vi "Teleop.vi"(10 "Match Info":T1={"Autonomous Elapsed Seconds"=0.0, "TeleOp Elapsed Seconds"=0.0, "Disabled Elapsed Seconds"=0.0, "Visited Autonomous"=FALSE, "Visited TeleOp"=FALSE, "Visited Disabled"=FALSE, "Autonomous Settings"={"Autonomous Style"=enum."Independent", "VI Refnum"=refnum}}, 11 "Call Context":T2) -> ()   [LabVIEW 2013]
doc: "This VI is called for each TeleOp packet received from the DS where the robot is not disabled. It is often used to read from the joysticks and update I/O or to update setpoints for timed control loops. It should complete and return within 20 milliseconds or it may miss DS packets."
uses:
  <vilib>/Rock Robotics/WPI/DriverStation/WPI_DriverStationDerivedRobotMode.ctl
  <vilib>/Rock Robotics/WPI/DriverStation/WPI_DriverStationMatch Info.ctl
  Robot Global Data.vi
  <vilib>/Rock Robotics/WPI/Joystick/WPI_JoystickGetSetRefNum.vi
  <vilib>/Rock Robotics/WPI/RobotDrive/WPI_RobotDriveGetSetRefNum.vi
panel:
  out "Numeric 1":dbl(slide) scale=0.0..100.0
  out "Boolean 2":bool
  out "Boolean 1":bool
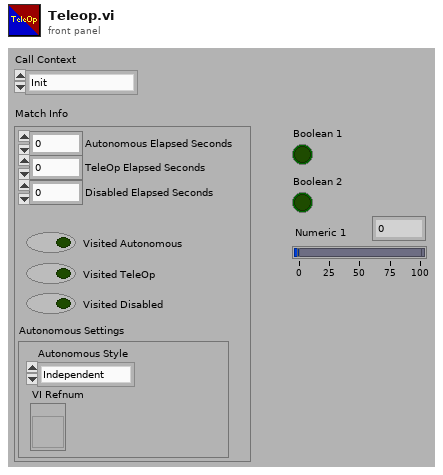
[diagram p1: front panel]
types:
  T1 = typedef "WPI_DriverStationMatch Info.ctl" = cluster{"Autonomous Elapsed Seconds":dbl, "TeleOp Elapsed Seconds":dbl, "Disabled Elapsed Seconds":dbl, "Visited Autonomous":bool, "Visited TeleOp":bool, "Visited Disabled":bool, "Autonomous Settings":cluster{"Autonomous Style":enum16{"Iterative", "Independent"}, "VI Refnum":refnum<vi>}}
  T2 = typedef "WPI_DriverStationDerivedRobotMode.ctl" = enum16{"Init", "Execute", "Stop"}
  T3 = typedef "WPI_JoystickDevRef.ctl" = cluster{"Device":T4}
  T4 = typedef "WPI_JoystickDeviceEnum.ctl" = enum16{"USB 1", "USB 2", "USB 3", "USB 4", "Kinect 1", "Kinect 2"}
  T5 = typedef "WPI_JoystickButtonState.ctl" = cluster{"Button 1":bool, "Button 2":bool, "Button 3":bool, "Button 4":bool, "Button 5":bool, "Button 6":bool, "Button 7":bool, "Button 8":bool, "Button 9":bool, "Button 10":bool, "Button 11":bool, "Button 12":bool}
  T6 = cluster{"axis 1 (x)":dbl, "axis 2 (y)":dbl, "axis 3 (throttle)":dbl, "axis 4":dbl, "axis 5":dbl, "axis 6":dbl}
  T7 = typedef "WPI_RobotDriveDevRef.ctl" = cluster{"DevStatus":errorcluster, "Motors[]":T8[], "Square Inputs":bool, "Max Output":dbl, "Isochronous":bool}
  T8 = typedef "WPI_MotorControlDeviceRef.ctl" = cluster{"DeviceStatus":errorcluster, "Type":enum16{"PWM", "CAN"}, "PWM":cluster{"Digital Module":T9, "PWM Channel":T10, "DeadBand":T11}, "CAN":cluster{"Device Number":u8, "Control Mode":T12, "Semaphore":T13, "Max Vout":dbl}, "Invert":bool, "TransformRef":T14, "InvTransformRef":T14}
  T9 = typedef "FPGA_TypedefDigitalModule.ctl" = enum16{"Digital Module 1", "Digital Module 2"}
  T10 = typedef "FPGA_DIOPWMChannel.ctl" = enum8{"PWM 1", "PWM 2", "PWM 3", "PWM 4", "PWM 5", "PWM 6", "PWM 7", "PWM 8", "PWM 9", "PWM 10", "Invalid"}
  T11 = typedef "WPI_PWMDeadband.ctl" = cluster{"Name":string, "maxPositivePwm":i32, "minPositivePwm":i32, "centerPwm":i32, "maxNegativePwm":i32, "minNegativePwm":i32, "angularRange":u16}
  T12 = typedef "WPI_CANJaguar_ControlMode.ctl" = enum8{"Percent VBus", "Current", "Speed", "Position", "Voltage"}
  T13 = typedef "Semaphore RefNum" = refnum<k1>
  T14 = typedef "WPI_PWMTransform_ConPane.ctl" = refnum<vi>
  T15 = typedef "WPI_ServoDeviceRef.ctl" = cluster{"DeviceStatus":errorcluster, "Digital Module":T9, "PWM Channel":T10, "DeadBand":T11}
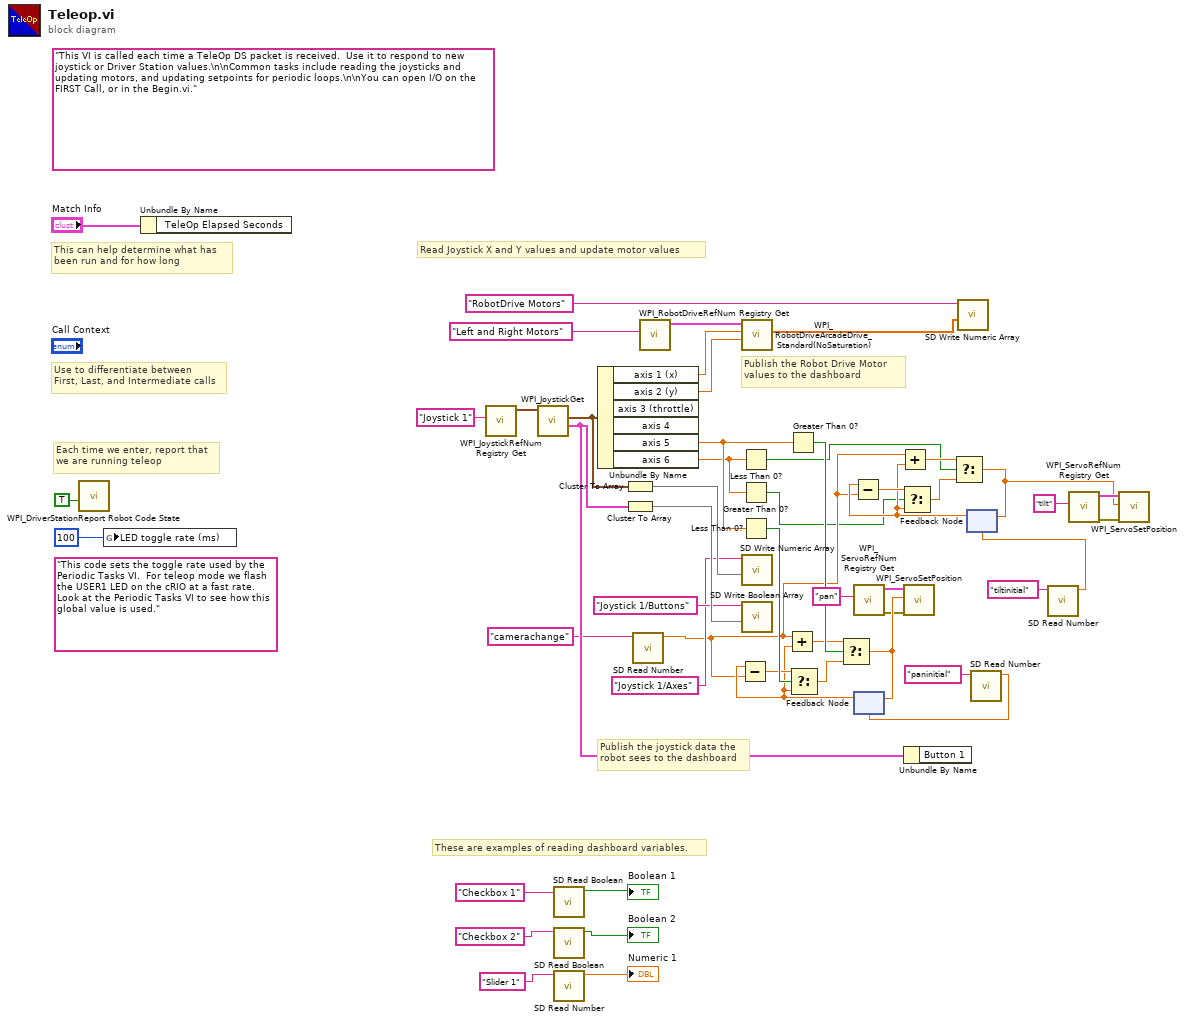
[diagram p0: block diagram]
diagram:
  (unwired) "This code sets the toggle rate used by the Periodic Tasks VI.  For teleop mode we flash the USER1 LED on the cRIO at a fast rate.  Look at the Periodic Tasks VI to see how this global value is used."
  (unwired) "This VI is called each time a TeleOp DS packet is received.  Use it to respond to new joystick or Driver Station values.\n\nCommon tasks include reading the joysticks and updating motors, and updating setpoints for periodic loops.\n\nYou can open I/O on the FIRST Call, or in the Begin.vi."
  # "These are examples of reading dashboard variables."
  # "Publish the Robot Drive Motor\nvalues to the dashboard"
  # "Publish the joystick data the\nrobot sees to the dashboard"
  # "Each time we enter, report that\nwe are running teleop"
  # "Use to differentiate between\nFirst, Last, and Intermediate calls"
  # "This can help determine what has\nbeen run and for how long"
  # "Read Joystick X and Y values and update motor values"
  n1 = call <vilib>:"WPI_DriverStationReport Robot Code State.vi"("TeleOp"=TRUE ("Autonomous")) -> ()  [unwired: 10 in, 1 out]
  n2 = global write "Robot Global Data.vi" "LED toggle rate (ms)"(u32 100 ("LED ms toggle rate")) -> ()
  n3 = Unbundle By Name("Match Info") -> ()  [unwired: 1 out]
  n4 = call <vilib>:"WPI_JoystickRefNum Registry Get.vi"("refnum name"="Joystick 1") -> ("JoystickDevRef"=w45:T3)  [unwired: 1 in, 9 out]
  n5 = call <vilib>:"WPI_JoystickGet.vi"("JoystickDevRef"=w45) -> ("Buttons"=w29:T5, "Axes"=w40:T6)  [unwired: 1 in, 4 out]
  n6 = call <vilib>:"SD Read Boolean.vi"("Name"="Checkbox 1" ("refnum name")) -> ("Boolean"=→"Boolean 1":bool)  [unwired: 8 in, 2 out]
  n7 = call <vilib>:"SD Read Boolean.vi"("Name"="Checkbox 2" ("refnum name")) -> ("Boolean"=→"Boolean 2":bool)  [unwired: 8 in, 2 out]
  n8 = call <vilib>:"SD Read Number.vi"("Name"="Slider 1" ("refnum name")) -> ("Numeric"=→"Numeric 1":dbl)  [unwired: 8 in, 2 out]
  n9 = Unbundle By Name(w40) -> ("axis 1 (x)"=w48:dbl, "axis 2 (y)"=w47:dbl, "axis 5"=w28:dbl, "axis 6"=w27:dbl)  [unwired: 2 out]
  n10 = Cluster To Array(cluster=w40) -> (array=w39:dbl[])
  n11 = Cluster To Array(cluster=w29) -> (array=w42:bool[])
  n12 = call <vilib>:"SD Read Number.vi"("Name"="camerachange") -> ("Numeric"=w8:dbl)  [unwired: 8 in, 2 out]
  n13 = call <vilib>:"WPI_RobotDriveRefNum Registry Get.vi"("refnum name"="Left and Right Motors") -> ("RobotDriveDevRef"=w49:T7)  [unwired: 1 in, 9 out]
  n14 = Less Than 0?(x=w27) -> (x < 0?=w7:bool)
  n15 = Greater Than 0?(x=w27) -> (x > 0?=w6:bool)
  n16 = Less Than 0?(x=w28) -> (x < 0?=w25:bool)
  n17 = call <vilib>:"WPI_RobotDriveArcadeDrive_Standard(NoSaturation).vi"("Y axis value"=w47, "X axis value"=w48, "RobotDriveDevRef"=w49) -> ("Motor Values"=w36:dbl[])  [unwired: 1 in, 7 out]
  n18 = call <vilib>:"SD Write Numeric Array.vi"("Numeric Array"=w39, "Name"="Joystick 1/Axes") -> ()  [unwired: 8 in, 2 out]
  n19 = call <vilib>:"SD Write Boolean Array.vi"("Boolean Array"=w42, "Name"="Joystick 1/Buttons") -> ()  [unwired: 8 in, 2 out]
  n20 = Greater Than 0?(x=w28) -> (x > 0?=w24:bool)
  n21 = call <vilib>:"WPI_ServoRefNum Registry Get.vi"("refnum name"="pan") -> ("error out"=w16:errorcluster, "ServoDeviceRef"=w17:T15)  [unwired: 9 in]
  n22 = Unbundle By Name(w29) -> ()  [unwired: 1 out]
  n23 = call <vilib>:"SD Write Numeric Array.vi"("Numeric Array"=w36, "Name"="RobotDrive Motors") -> ()  [unwired: 8 in, 2 out]
  n24 = call <vilib>:"SD Read Number.vi"("Name"="paninitial") -> ("Numeric"=w3:dbl)  [unwired: 8 in, 2 out]
  n25 = feedback #1(w3) -> (w19:dbl)
  n26 = Subtract(x=w19, y=w8) -> (x-y=w21:dbl)
  n27 = Add(x=w8, y=w19) -> (x+y=w20:dbl)
  n28 = Select(t=w21, s=w25, f=w19) -> (s? t:f=w22:dbl)
  n29 = Select(t=w20, s=w24, f=w22) -> (s? t:f=w23:dbl)
  n30 = feedback-in #1(w23) -> ()
  n31 = call <vilib>:"WPI_ServoSetPosition.vi"("error in (no error)"=w16, "Position"=w23, "ServoDeviceRef"=w17) -> ()  [unwired: 7 in, 2 out]
  n32 = call <vilib>:"SD Read Number.vi"("Name"="tiltinitial") -> ("Numeric"=w4:dbl)  [unwired: 8 in, 2 out]
  n33 = feedback #2(w4) -> (w12:dbl)
  n34 = Subtract(x=w12, y=w8) -> (x-y=w14:dbl)
  n35 = Add(x=w8, y=w12) -> (x+y=w13:dbl)
  n36 = Select(t=w14, s=w6, f=w12) -> (s? t:f=w15:dbl)
  n37 = Select(t=w13, s=w7, f=w15) -> (s? t:f=w5:dbl)
  n38 = feedback-in #2(w5) -> ()
  n39 = call <vilib>:"WPI_ServoRefNum Registry Get.vi"("refnum name"="tilt") -> ("error out"=w9:errorcluster, "ServoDeviceRef"=w10:T15)  [unwired: 9 in]
  n40 = call <vilib>:"WPI_ServoSetPosition.vi"("error in (no error)"=w9, "Position"=w5, "ServoDeviceRef"=w10) -> ()  [unwired: 7 in, 2 out]
